vi "bangBangPlanning.vi"(0 "Game in":refnum<class "Game.lvclass">, 1 "array":dbl[][](array[numeric]), 2 "est_vtang":dbl, 3 "desired_vtang":dbl, 4 "delta":dbl, 5 "error in (no error)":errorcluster, 6 "v_max":dbl=4.0, 7 "dist_to_dest":dbl=2000.0) -> (14 "Game out":refnum<class "Game.lvclass">, 19 "error out":errorcluster)   [LabVIEW 2020, in "Game.lvclass"]
uses:
  Game.lvclass
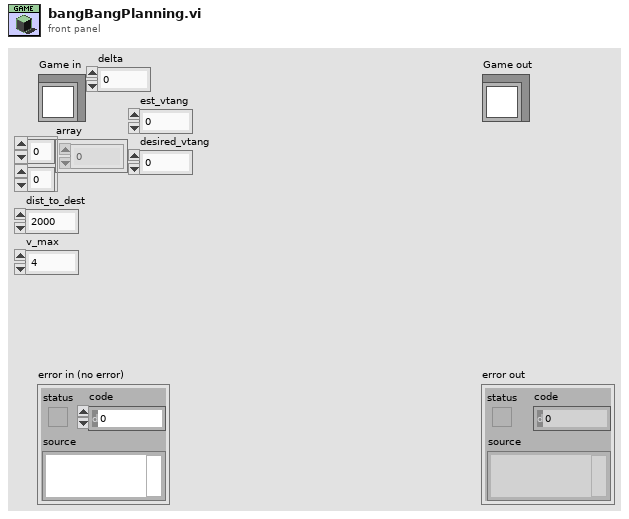
[diagram p1: front panel]
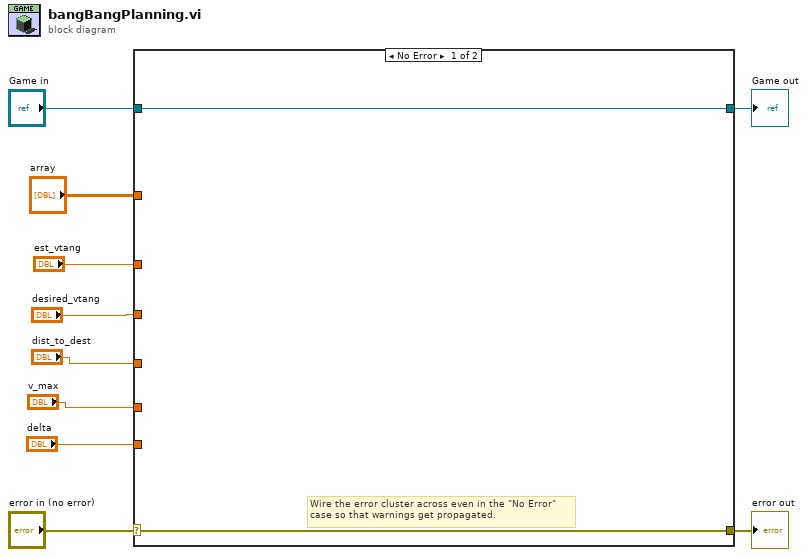
[diagram p0: block diagram]
diagram:
  n1 = case shown="No Error" "error in (no error)" {
    selector: "error in (no error)" -> [w11 w14]
    tunnel: [w11 w14] -> w9
    tunnel: [w12 w13] -> w7
    tunnel: "Game in" -> [w12 w13]
    tunnel: "array" -> [_ _]
    tunnel: "est_vtang" -> [_ _]
    tunnel: "desired_vtang" -> [_ _]
    tunnel: "delta" -> [_ _]
    tunnel: "dist_to_dest" -> [_ _]
    tunnel: "v_max" -> [_ _]
    frame No Error {
      # "Wire the error cluster across even in the \"No Error\"\ncase so that warnings get propagated."
    }
    frame Error {
    }
  }
  "error out" <- w9
  "Game out" <- w7
